vi "1D To 2D.vi"(7 "1D Pixel Data in":u32[](array[numeric]), 11 "2D Pixel Data in":u32[][](array[numeric])) -> (3 "2D Pixel Data out":u32[][](array[numeric]))   [LabVIEW 2020, in "3D.lvlib"]
uses:
  3D.lvlib
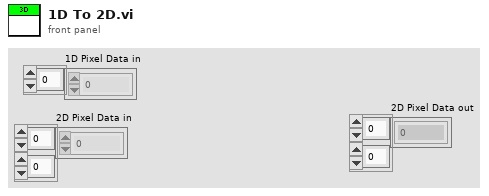
[diagram p1: front panel]
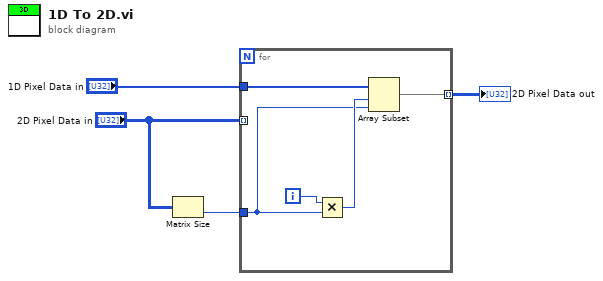
[diagram p0: block diagram]
diagram:
  n1 = Matrix Size(0:"2D Pixel Data in") -> (2:w1:i32)  [unwired: 1 out]
  n2 = for {
    tunnel: "2D Pixel Data in" -> [_] mode=indexing
    tunnel: "1D Pixel Data in" -> [w9]
    tunnel: [w8] -> w3 mode=indexing
    tunnel: w1 -> [w5]
    i -> [w7]
    n3 = Multiply(x=w7, y=w5) -> (x*y=w6:i32)
    n4 = Array Subset(array=w9, index=w6, length=w5) -> (w8:u32[])
  }
  "2D Pixel Data out" <- w3
